vi "ReadPersistentConfiguration.vi"(8 "Error In":errorcluster, 10 "DataIn":variant, 11 "OpenCVFaceDetection in":refnum<class "OpenCVFaceDetection.lvclass">) -> (0 "Error Out":errorcluster, 2 "DataOut":variant, 3 "OpenCVFaceDetection out":refnum<class "OpenCVFaceDetection.lvclass">)   [LabVIEW 2021, in "OpenCVFaceDetection.lvclass"]
uses:
  OpenCVFaceDetection.lvclass
  OpenCVFaceDetection.lvclass/OpenCVFaceDetection.ctl
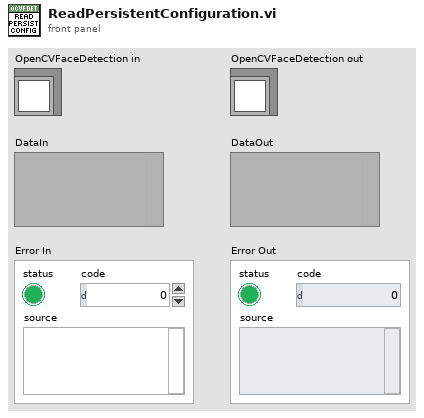
[diagram p1: front panel]
types:
  T1 = cluster{"scaleFactor":dbl, "minNeighbors":i32, "Color":dbl, "Size":cluster{"height":i32, "width":i32}}
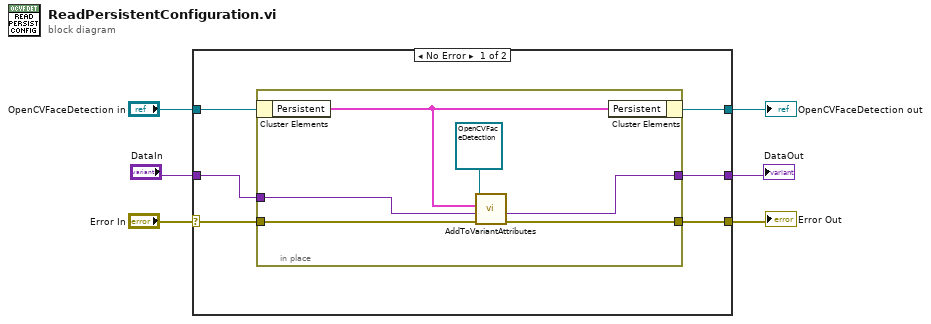
[diagram p0: block diagram]
diagram:
  n1 = case shown="No Error" "Error In" {
    selector: "Error In" -> [w10 w21]
    tunnel: [w9 w21] -> w5
    tunnel: [w7 w20] -> w3
    tunnel: "OpenCVFaceDetection in" -> [w12 w20]
    tunnel: "DataIn" -> [w11 w19]
    tunnel: [w8 w19] -> w1
    frame No Error {
      n2 = in-place {
        in-place-border: [w17] -> w9
        in-place-border: w11 -> [w16]
        in-place-border: [w15] -> w8
        in-place-border: w10 -> [w18]
        n3 = in-place-cluster #1(w12) -> ("Persistent"=w13:T1)
        n4 = call "AddToVariantAttributes.vi"("error in (no error)"=w18, "DataIn in"=w16, "PersistentData"=w13, "Object"=refnum<class "OpenCVFaceDetection.lvclass"> refnum ("ApplicationGUI2")) -> ("error out"=w17:errorcluster, "DataIn out"=w15:variant)  [unwired: 6 in]
        n5 = in-place-cluster #1("Persistent"=w13) -> (w7:refnum<class "OpenCVFaceDetection.lvclass">)
      }
    }
    frame Error {
    }
  }
  "Error Out" <- w5
  "OpenCVFaceDetection out" <- w3
  "DataOut" <- w1
